vi "Close.vi"(8 "error in (no error)":errorcluster, 11 "Fetch 10kHz in":refnum<class "Continuous Waveform Acq CFG.lvclass">) -> (0 "error out":errorcluster, 3 "Fetch 10kHz out":refnum<class "Continuous Waveform Acq CFG.lvclass">)   [LabVIEW 2023, in "PXIe-5172 Simulated.lvlib" / "Continuous Waveform Acq CFG.lvclass"]
uses:
  Continuous Waveform Acq CFG.lvclass
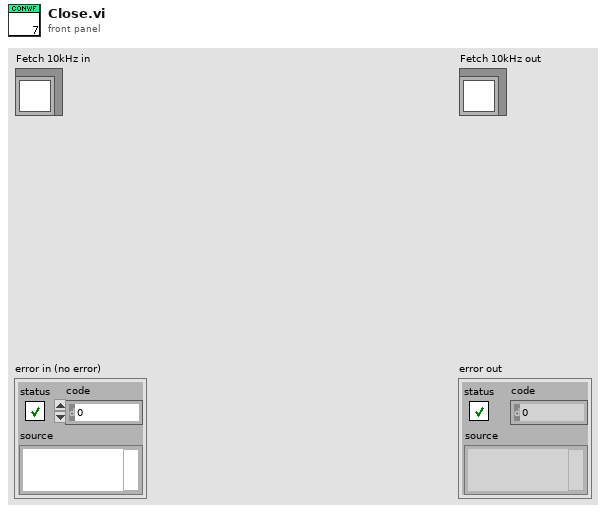
[diagram p1: front panel]
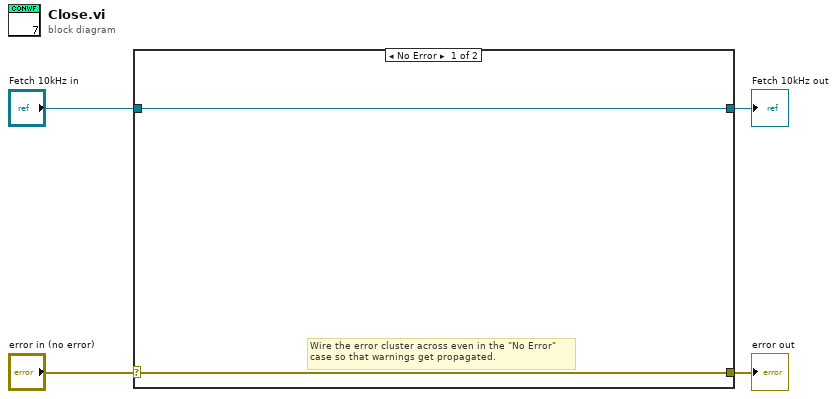
[diagram p0: block diagram]
diagram:
  n1 = case shown="No Error" "error in (no error)" {
    selector: "error in (no error)" -> [w5 w8]
    tunnel: [w5 w8] -> w3
    tunnel: [w6 w7] -> w1
    tunnel: "Fetch 10kHz in" -> [w6 w7]
    frame No Error {
      # "Wire the error cluster across even in the \"No Error\"\ncase so that warnings get propagated."
    }
    frame Error {
    }
  }
  "error out" <- w3
  "Fetch 10kHz out" <- w1
